vi "Simple Add.vi"(9 "y":dbl, 11 "x":dbl) -> (3 "x+y+z":dbl)   [LabVIEW 2017]
panel:
  in  "z 2":dbl
  in  "z":dbl
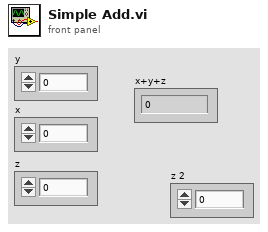
[diagram p1: front panel]
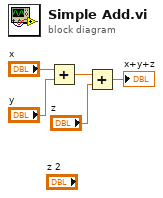
[diagram p0: block diagram]
diagram:
  n1 = Add(x="x", y="y") -> (x+y=w3:dbl)
  n2 = Add(x=w3, y="z") -> (x+y=→"x+y+z":dbl)
